vi "InitBaseMission.vi"(10 "Boat Location":refnum<notifier>, 11 "Mission Notifiers":T1) -> (3 "Mission Notifiers OUT":T1)   [LabVIEW 2013]
doc: "This VI initializes a base mission (Idle at point) at the indicated boat position. Unimplemented possibilities:\n1) Choose the desired idle point at the beeginning\n2) Idle where the boat starts\nThis VI was mostly created to clean up Forebrain Main.\n\nEric Schneider, August 2014"
uses:
  Data/TypeDefs/UTM Location.ctl
  Data/TypeDefs/MissionNotifiers.ctl
  Classes/Missions/GenericMission/GenericMission.lvclass
  Classes/Obstacle/Obstacle.lvclass
  Classes/Missions/Idle/Idle.lvclass
  Data/TypeDefs/MissionTypeControl.ctl
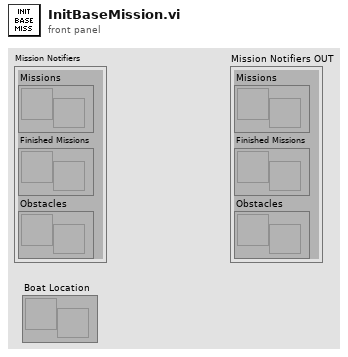
[diagram p1: front panel]
types:
  T1 = typedef "MissionNotifiers.ctl" = cluster{"Missions":refnum<notifier>, "Finished Missions":refnum<notifier>, "Obstacles":refnum<notifier>}
  T2 = typedef "MissionTypeControl.ctl" = enum16{"Idle at Point", "Drive to Waypoint", "Round Buoy to Port", "Round Buoy to Starboard", "Pass Between Buoys", "Station Keeping"}
  T3 = typedef "UTM Location.ctl" = cluster{"UTM Zone":dbl, "Hemisphere":enum16{"North", "South"}, "East":dbl, "North":dbl}
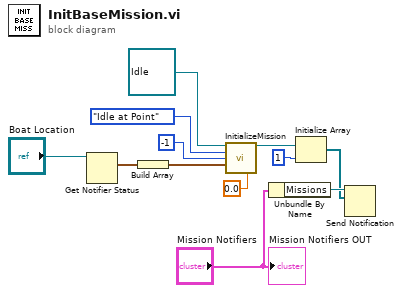
[diagram p0: block diagram]
diagram:
  n1 = Get Notifier Status(notifier="Boat Location") -> (current notification=w8:T3)  [unwired: 1 in, 4 out]
  n2 = Build Array(w8) -> (w9:T3[])
  n3 = call-dynamic "InitializeMission.vi"("GenericMission in"=refnum<class "Idle.lvclass"> refnum ("Idle.lvclass"), "Mission Type"=MissionTypeControl."Idle at Point", "ID#"=i16 -1, "Points of Interest"=w9, "Tolerance (m)"=0.0) -> ("GenericMission out"=w6:refnum<class "Idle.lvclass">)  [unwired: 9 in, 1 out]
  n4 = Unbundle By Name("Mission Notifiers") -> ("Missions"=w2:refnum<notifier>)
  n5 = Initialize Array(w6, 1 ("dimension size")) -> (w1:refnum<class "Idle.lvclass">[])
  n6 = Send Notification(notification=w1, notifier=w2) -> ()  [unwired: 1 in, 2 out]
  "Mission Notifiers OUT" <- "Mission Notifiers"
